vi "Write State.vi"(8 "error in (no error)":errorcluster, 10 "Enum":T1, 11 "Cargo in":refnum<class "Cargo.lvclass">) -> (0 "error out":errorcluster, 3 "Cargo out":refnum<class "Cargo.lvclass">)   [LabVIEW 2018, in "Cargo.lvlib" / "Cargo.lvclass"]
uses:
  Cargo.lvclass
  Controls/Cargo States.ctl
  Cargo.lvclass/Cargo.ctl
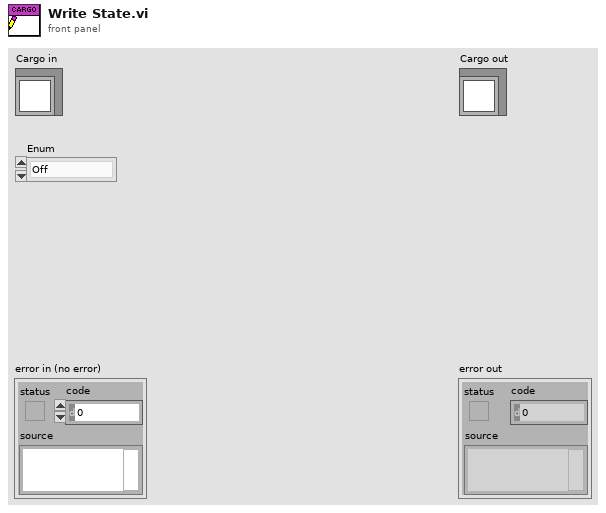
[diagram p1: front panel]
types:
  T1 = typedef "Cargo.lvlib/Cargo.lvclass/Cargo States.ctl" = enum16{"Off", "Intake Full", "Intake Idle", "Output Full"}
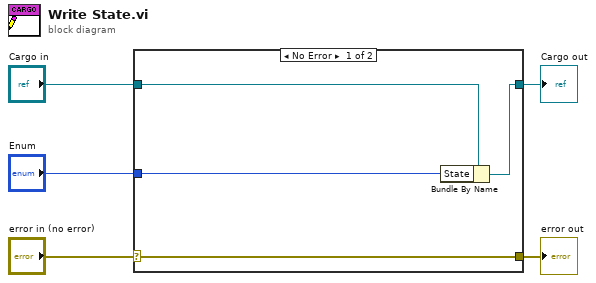
[diagram p0: block diagram]
diagram:
  n1 = case shown="No Error" "error in (no error)" {
    selector: "error in (no error)" -> [w9 w10]
    tunnel: [w9 w10] -> w4
    tunnel: [w7 w11] -> w2
    tunnel: "Cargo in" -> [w8 w11]
    tunnel: "Enum" -> [w6 _]
    frame No Error {
      n2 = Bundle By Name(cluster=w8, "State"=w6) -> (w7:refnum<class "Cargo.lvclass">)
    }
    frame Error {
    }
  }
  "error out" <- w4
  "Cargo out" <- w2
